vi "MatrixSwitch.vi"(8 "error in (no error)":errorcluster, 10 "Action":T1(ring), 11 "GPIBSwitching in":refnum<class "GPIBSwitching.lvclass">) -> (0 "error out":errorcluster, 3 "GPIBSwitching out":refnum<class "GPIBSwitching.lvclass">)   [LabVIEW 2018, in "GPIBSwitching.lvclass"]
uses:
  GPIBSwitching.lvclass
  InstrumentSetup.vi
  InstrControl.lvclass
panel:
  out "Display Matrix":bool[][](array[boolean])
  # "Pickering Matrix Settings"
  # "X1"
  # "X2"
  # "X3"
  # "X4"
  # "X5"
  # "X6"
  # "X7"
  # "X8"
  # "X9"
  # "X10"
  # "X11"
  # "X12"
  # "Y1"
  # "Y2"
  # "Y3"
  # "Y4"
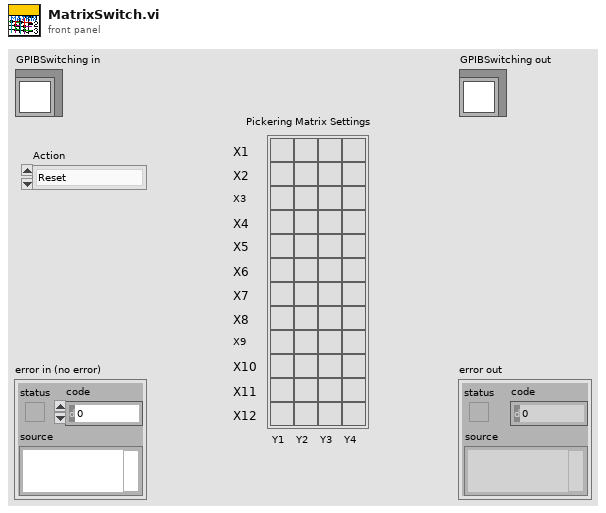
[diagram p1: front panel]
types:
  T1 = enum16{"Reset", "Ground", "Striptest SMU", "Striptest LCR", "IV", "CV", "Interstrip Cap", "Interstrip Res", "Setup StripTest"}
  T2 = cluster{"Matrix address":string, "Mux1 address":string, "Mux2 address":string, "Matrix used?":bool, "Switching":refnum<class "Switching.lvclass">, "Matrix X Channels":cluster{"Bias Supply / SMU LO":i32, "Bias Supply / SMU HI":i32, "CV Box LO":i32, "CV Box HI":i32, "CV Box LO IN":i32, "CV Box HI IN":i32, "Volt meter LO":i32, "Volt meter HI":i32, "Mux1 C1":i32, "Mux1 C2":i32, "Mux2 C1":i32, "Mux2 C2":i32}}
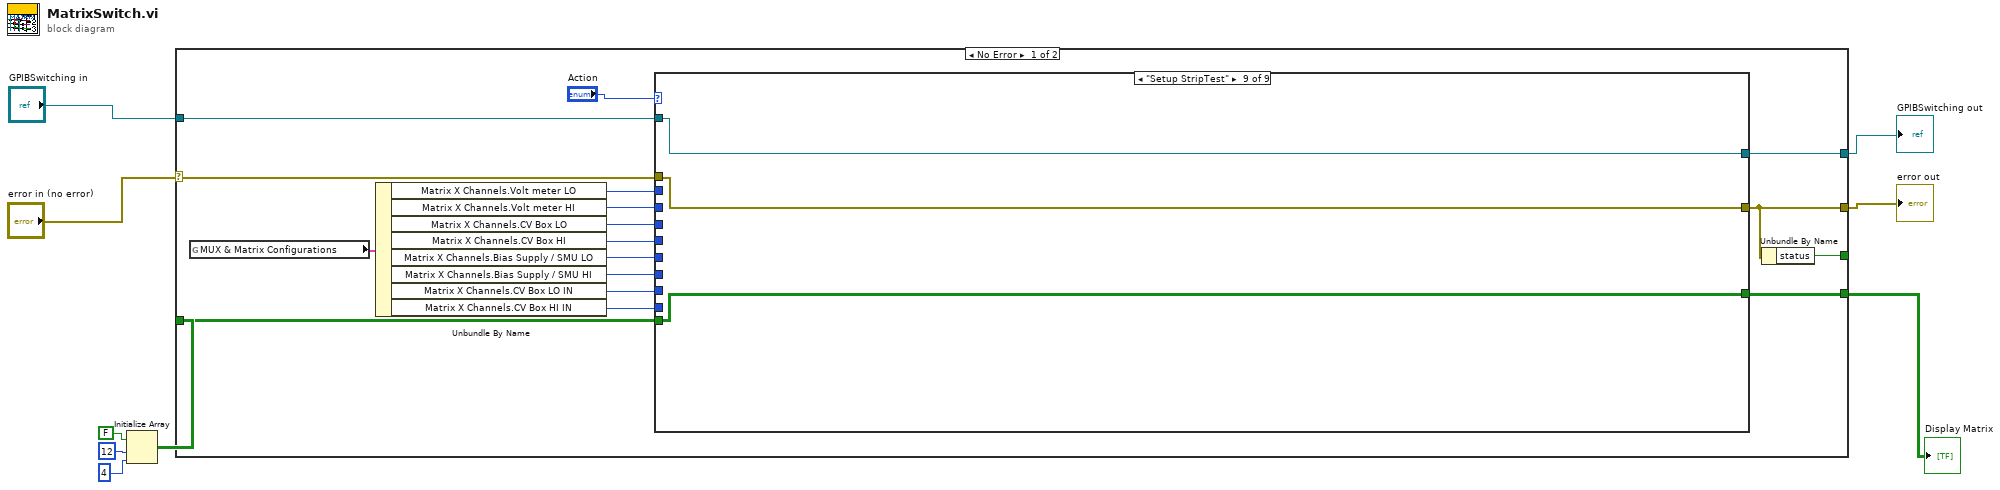
[diagram p0: block diagram]
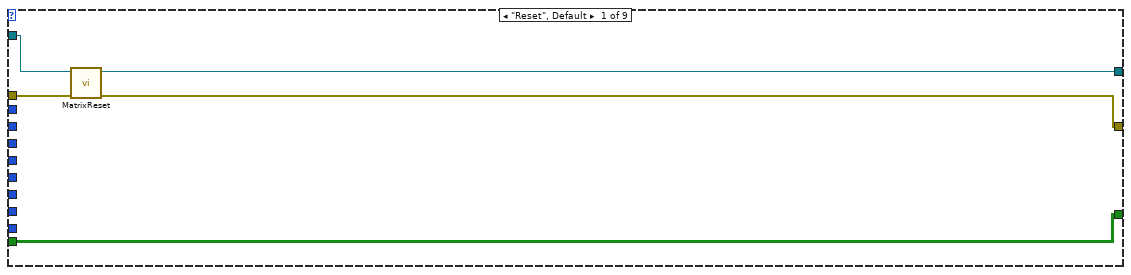
[diagram p2: hidden frame]
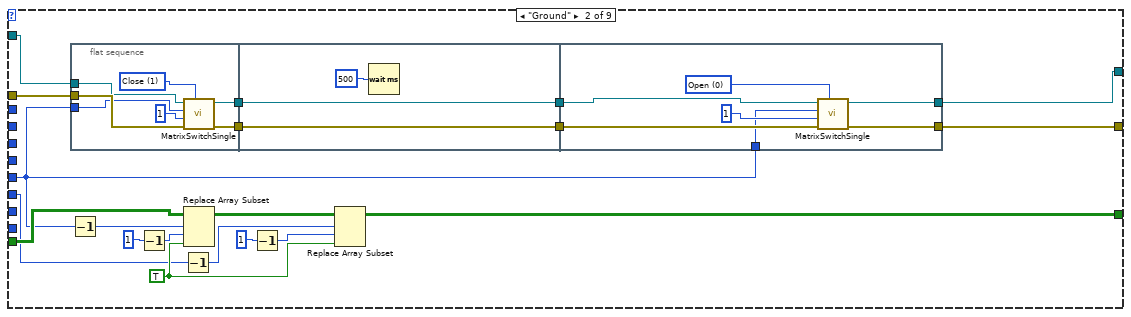
[diagram p3: hidden frame]
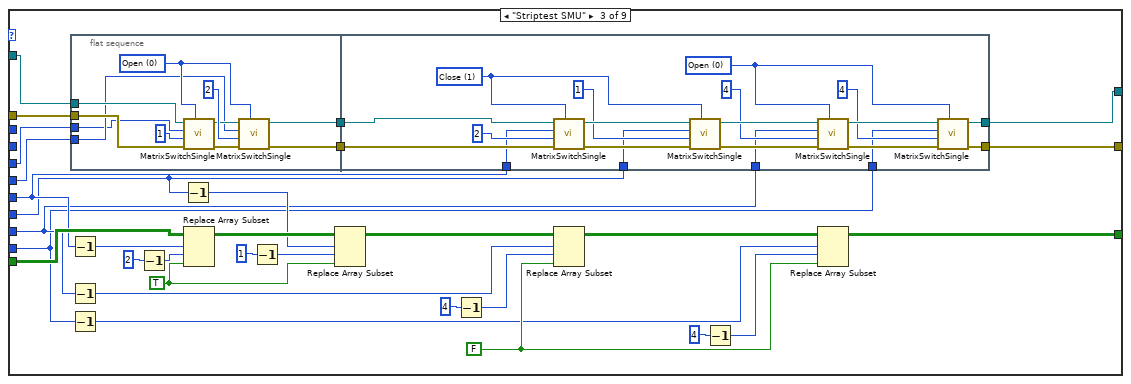
[diagram p4: hidden frame]
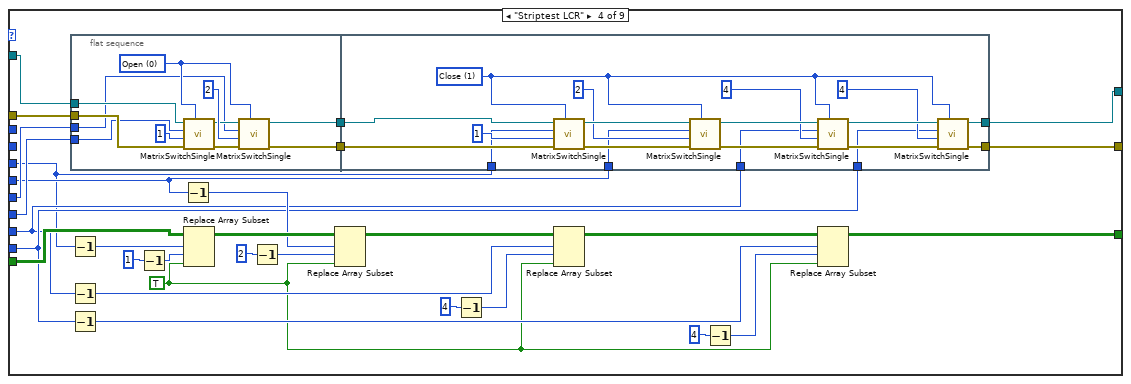
[diagram p5: hidden frame]
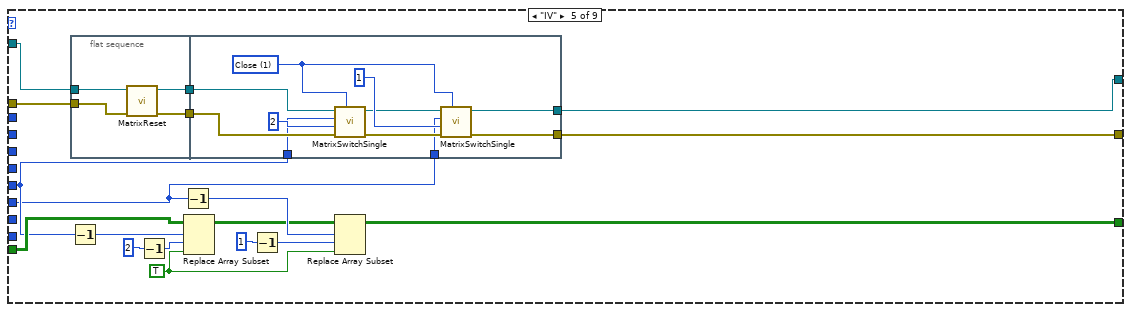
[diagram p6: hidden frame]
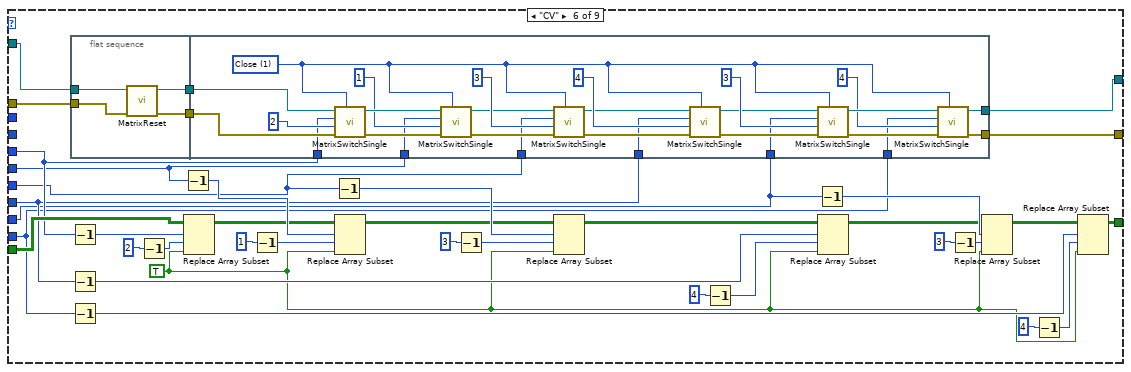
[diagram p7: hidden frame]
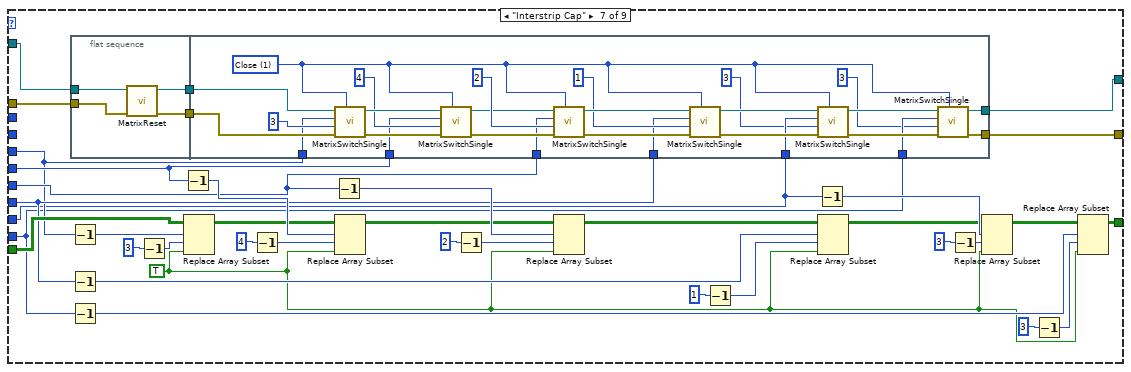
[diagram p8: hidden frame]
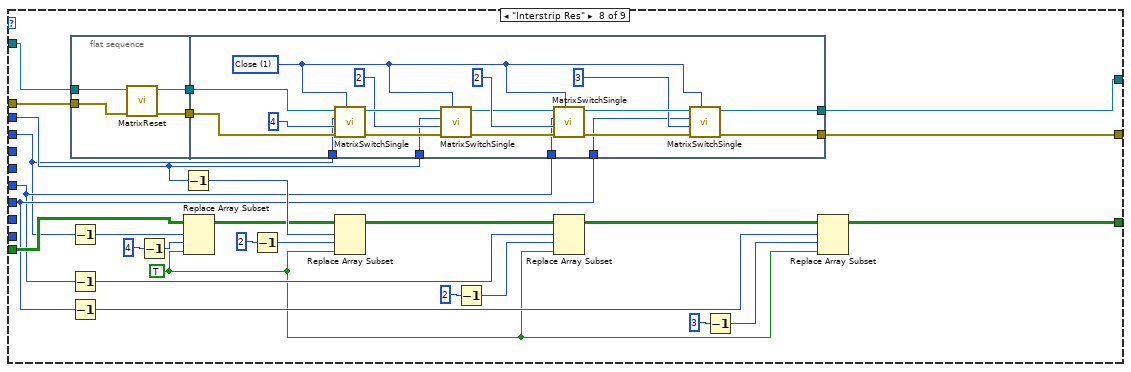
[diagram p9: hidden frame]
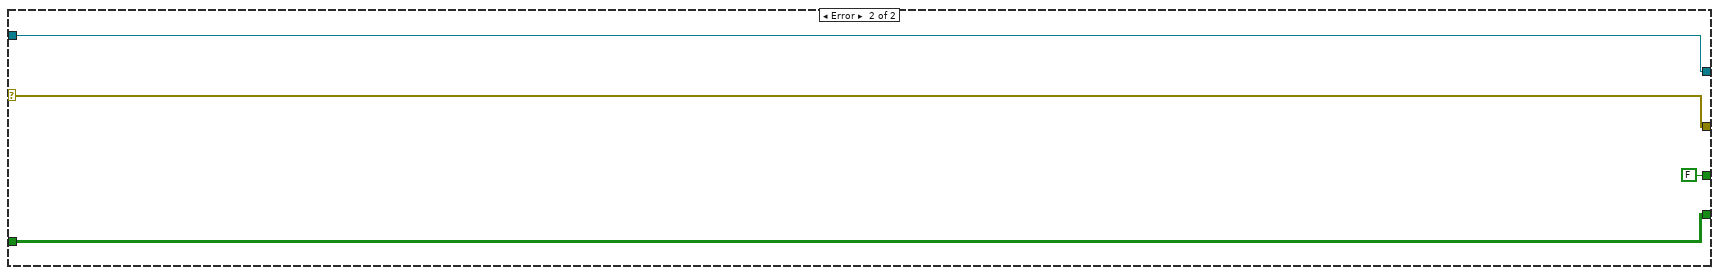
[diagram p10: hidden frame]
diagram:
  n1 = Initialize Array(FALSE, 12, 4) -> (w5:bool[][])
  n2 = case shown="No Error" "error in (no error)" {
    selector: "error in (no error)" -> [w20 w419]
    tunnel: [w23 w419] -> w3
    tunnel: [w24 w418] -> w4
    tunnel: "GPIBSwitching in" -> [w21 w418]
    tunnel: [w22 FALSE] -> _
    tunnel: w5 -> [w26 w416]
    tunnel: [w25 w416] -> w9
    frame No Error {
      n3 = global read "InstrumentSetup.vi" "MUX & Matrix Configurations"() -> (w19:T2)
      n4 = Unbundle By Name(w19) -> ("Matrix X Channels.Volt meter LO"=w13:i32, "Matrix X Channels.Volt meter HI"=w14:i32, "Matrix X Channels.CV Box LO"=w18:i32, "Matrix X Channels.CV Box HI"=w17:i32, "Matrix X Channels.Bias Supply / SMU LO"=w11:i32, "Matrix X Channels.Bias Supply / SMU HI"=w12:i32, "Matrix X Channels.CV Box LO IN"=w16:i32, "Matrix X Channels.CV Box HI IN"=w15:i32)
      n5 = case shown="\"Setup StripTest\"" "Action" {
        tunnel: w26 -> [w31 w36 w86 w149 w199 w236 w316 w374 w413]
        tunnel: [w31 w34 w85 w148 w200 w237 w293 w375 w413] -> w25
        tunnel: w20 -> [w28 w51 w75 w138 w207 w235 w315 w373 w414]
        tunnel: w21 -> [w30 w48 w77 w137 w208 w234 w314 w372 w415]
        tunnel: [w29 w45 w80 w143 w196 w230 w310 w368 w415] -> w24
        tunnel: [w27 w44 w79 w142 w195 w231 w311 w369 w414] -> w23
        tunnel: w11 -> [_ w33 w72 w135 w192 w227 w307 w364 _]
        tunnel: w12 -> [_ w32 w71 w136 w191 w226 w308 w365 _]
        tunnel: w18 -> [_ _ w73 w131 _ w229 w305 _ _]
        tunnel: w17 -> [_ _ w74 w132 _ w228 w306 _ _]
        tunnel: w16 -> [_ _ w70 w133 _ w225 w297 _ _]
        tunnel: w15 -> [_ _ w69 w134 _ w224 w296 _ _]
        tunnel: w13 -> [_ _ _ _ _ _ _ w363 _]
        tunnel: w14 -> [_ _ _ _ _ _ _ w362 _]
        frame "Reset", Default {
          n6 = call-dynamic "MatrixReset.vi"("error in (no error)"=w28, "GPIBSwitching in"=w30) -> ("error out"=w27:errorcluster, "GPIBSwitching out"=w29:refnum<class "GPIBSwitching.lvclass">)  [unwired: 8 in]
        }
        frame "Ground" {
          w42 = TRUE
          n7 = Decrement(x=w33) -> (x-1=w37:i32)
          n8 = flat-sequence {
            tunnel: w51 -> [w56]
            tunnel: [w55] -> w50
            tunnel: w48 -> [w54]
            tunnel: [w53] -> w46
            tunnel: w33 -> [w52]
            tunnel: w50 -> [w60]
            tunnel: [w60] -> w49
            tunnel: [w59] -> w47
            tunnel: w46 -> [w59]
            tunnel: w49 -> [w67]
            tunnel: w47 -> [w65]
            tunnel: [w64] -> w45
            tunnel: [w63] -> w44
            tunnel: w33 -> [w62]
            frame #0 {
              w58 = u16 1 items=["Open", "Close"] ("Switch action")
              n9 = call-dynamic "MatrixSwitchSingle.vi"("Switch action"=w58, "error in (no error)"=w56, "Matrix Y"=1, "Matrix X"=w52, "GPIBSwitching in"=w54) -> ("error out"=w55:errorcluster, "GPIBSwitching out"=w53:refnum<class "GPIBSwitching.lvclass">)  [unwired: 4 in, 1 out]
            }
            frame #1 {
              n10 = Wait (ms)(milliseconds to wait=u32 500) -> ()  [unwired: 1 out]
            }
            frame #2 {
              w68 = u16 0 items=["Open", "Close"] ("Switch action")
              n11 = call-dynamic "MatrixSwitchSingle.vi"("Switch action"=w68, "error in (no error)"=w67, "Matrix Y"=1, "Matrix X"=w62, "GPIBSwitching in"=w65) -> ("error out"=w63:errorcluster, "GPIBSwitching out"=w64:refnum<class "GPIBSwitching.lvclass">)  [unwired: 4 in, 1 out]
            }
          }
          n12 = Decrement(x=1 ("Matrix Y")) -> (x-1=w38:i32)
          n13 = Decrement(x=w32) -> (x-1=w39:i32)
          n14 = Replace Array Subset(array=w36, new element=w42, index (row)=w37, index (col)=w38) -> (w43:bool[][])
          n15 = Decrement(x=1 ("Matrix Y")) -> (x-1=w40:i32)
          n16 = Replace Array Subset(array=w43, new element=w42, index (row)=w39, index (col)=w40) -> (w34:bool[][])
        }
        frame "Striptest SMU" {
          w99 = FALSE
          w98 = TRUE
          n17 = Decrement(x=w72) -> (x-1=w88:i32)
          n18 = Decrement(x=w70) -> (x-1=w93:i32)
          n19 = Decrement(x=w69) -> (x-1=w94:i32)
          n20 = flat-sequence {
            tunnel: [w106] -> w78
            tunnel: w77 -> [w104]
            tunnel: [w103] -> w76
            tunnel: w75 -> [w102]
            tunnel: w74 -> [w101]
            tunnel: w73 -> [w100]
            tunnel: [w119] -> w80
            tunnel: [w118] -> w79
            tunnel: w78 -> [w116]
            tunnel: w76 -> [w115]
            tunnel: w70 -> [w114]
            tunnel: w69 -> [w113]
            tunnel: w71 -> [w112]
            tunnel: w72 -> [w111]
            frame #0 {
              w105 = u16 0 items=["Open", "Close"] ("Switch action")
              n21 = call-dynamic "MatrixSwitchSingle.vi"("Switch action"=w105, "error in (no error)"=w102, "Matrix Y"=1, "Matrix X"=w100, "GPIBSwitching in"=w104) -> ("error out"=w109:errorcluster, "GPIBSwitching out"=w108:refnum<class "GPIBSwitching.lvclass">)  [unwired: 4 in, 1 out]
              n22 = call-dynamic "MatrixSwitchSingle.vi"("Switch action"=w105, "error in (no error)"=w109, "Matrix Y"=2, "Matrix X"=w101, "GPIBSwitching in"=w108) -> ("error out"=w106:errorcluster, "GPIBSwitching out"=w103:refnum<class "GPIBSwitching.lvclass">)  [unwired: 4 in, 1 out]
            }
            frame #1 {
              w117 = u16 0 items=["Open", "Close"] ("Switch action")
              w128 = u16 1 items=["Open", "Close"] ("Switch action")
              n23 = call-dynamic "MatrixSwitchSingle.vi"("Switch action"=w128, "error in (no error)"=w116, "Matrix Y"=2, "Matrix X"=w111, "GPIBSwitching in"=w115) -> ("error out"=w126:errorcluster, "GPIBSwitching out"=w129:refnum<class "GPIBSwitching.lvclass">)  [unwired: 4 in, 1 out]
              n24 = call-dynamic "MatrixSwitchSingle.vi"("Switch action"=w128, "error in (no error)"=w126, "Matrix Y"=1, "Matrix X"=w112, "GPIBSwitching in"=w129) -> ("error out"=w124:errorcluster, "GPIBSwitching out"=w125:refnum<class "GPIBSwitching.lvclass">)  [unwired: 4 in, 1 out]
              n25 = call-dynamic "MatrixSwitchSingle.vi"("Switch action"=w117, "error in (no error)"=w124, "Matrix Y"=4, "Matrix X"=w114, "GPIBSwitching in"=w125) -> ("error out"=w121:errorcluster, "GPIBSwitching out"=w122:refnum<class "GPIBSwitching.lvclass">)  [unwired: 4 in, 1 out]
              n26 = call-dynamic "MatrixSwitchSingle.vi"("Switch action"=w117, "error in (no error)"=w121, "Matrix Y"=4, "Matrix X"=w113, "GPIBSwitching in"=w122) -> ("error out"=w118:errorcluster, "GPIBSwitching out"=w119:refnum<class "GPIBSwitching.lvclass">)  [unwired: 4 in, 1 out]
            }
          }
          n27 = Decrement(x=2 ("Matrix Y")) -> (x-1=w87:i32)
          n28 = Decrement(x=w71) -> (x-1=w89:i32)
          n29 = Replace Array Subset(array=w86, new element=w98, index (row)=w88, index (col)=w87) -> (w91:bool[][])
          n30 = Decrement(x=1 ("Matrix Y")) -> (x-1=w90:i32)
          n31 = Replace Array Subset(array=w91, new element=w98, index (row)=w89, index (col)=w90) -> (w97:bool[][])
          n32 = Decrement(x=4 ("Matrix Y")) -> (x-1=w92:i32)
          n33 = Replace Array Subset(array=w97, new element=w99, index (row)=w93, index (col)=w92) -> (w96:bool[][])
          n34 = Decrement(x=4 ("Matrix Y")) -> (x-1=w95:i32)
          n35 = Replace Array Subset(array=w96, new element=w99, index (row)=w94, index (col)=w95) -> (w85:bool[][])
        }
        frame "Striptest LCR" {
          w141 = TRUE
          n36 = Decrement(x=w131) -> (x-1=w151:i32)
          n37 = Decrement(x=w133) -> (x-1=w156:i32)
          n38 = Decrement(x=w134) -> (x-1=w157:i32)
          n39 = flat-sequence {
            tunnel: [w167] -> w140
            tunnel: [w166] -> w139
            tunnel: w138 -> [w165]
            tunnel: w137 -> [w164]
            tunnel: w135 -> [w162]
            tunnel: w136 -> [w161]
            tunnel: [w180] -> w143
            tunnel: [w179] -> w142
            tunnel: w140 -> [w177]
            tunnel: w139 -> [w176]
            tunnel: w131 -> [w175]
            tunnel: w132 -> [w174]
            tunnel: w133 -> [w173]
            tunnel: w134 -> [w172]
            frame #0 {
              w163 = u16 0 items=["Open", "Close"] ("Switch action")
              n40 = call-dynamic "MatrixSwitchSingle.vi"("Switch action"=w163, "error in (no error)"=w165, "Matrix Y"=1, "Matrix X"=w161, "GPIBSwitching in"=w164) -> ("error out"=w170:errorcluster, "GPIBSwitching out"=w169:refnum<class "GPIBSwitching.lvclass">)  [unwired: 4 in, 1 out]
              n41 = call-dynamic "MatrixSwitchSingle.vi"("Switch action"=w163, "error in (no error)"=w170, "Matrix Y"=2, "Matrix X"=w162, "GPIBSwitching in"=w169) -> ("error out"=w166:errorcluster, "GPIBSwitching out"=w167:refnum<class "GPIBSwitching.lvclass">)  [unwired: 4 in, 1 out]
            }
            frame #1 {
              w178 = u16 1 items=["Open", "Close"] ("Switch action")
              n42 = call-dynamic "MatrixSwitchSingle.vi"("Switch action"=w178, "error in (no error)"=w176, "Matrix Y"=1, "Matrix X"=w175, "GPIBSwitching in"=w177) -> ("error out"=w187:errorcluster, "GPIBSwitching out"=w189:refnum<class "GPIBSwitching.lvclass">)  [unwired: 4 in, 1 out]
              n43 = call-dynamic "MatrixSwitchSingle.vi"("Switch action"=w178, "error in (no error)"=w187, "Matrix Y"=2, "Matrix X"=w174, "GPIBSwitching in"=w189) -> ("error out"=w185:errorcluster, "GPIBSwitching out"=w186:refnum<class "GPIBSwitching.lvclass">)  [unwired: 4 in, 1 out]
              n44 = call-dynamic "MatrixSwitchSingle.vi"("Switch action"=w178, "error in (no error)"=w185, "Matrix Y"=4, "Matrix X"=w173, "GPIBSwitching in"=w186) -> ("error out"=w182:errorcluster, "GPIBSwitching out"=w183:refnum<class "GPIBSwitching.lvclass">)  [unwired: 4 in, 1 out]
              n45 = call-dynamic "MatrixSwitchSingle.vi"("Switch action"=w178, "error in (no error)"=w182, "Matrix Y"=4, "Matrix X"=w172, "GPIBSwitching in"=w183) -> ("error out"=w179:errorcluster, "GPIBSwitching out"=w180:refnum<class "GPIBSwitching.lvclass">)  [unwired: 4 in, 1 out]
            }
          }
          n46 = Decrement(x=1 ("Matrix Y")) -> (x-1=w150:i32)
          n47 = Decrement(x=w132) -> (x-1=w152:i32)
          n48 = Replace Array Subset(array=w149, new element=w141, index (row)=w151, index (col)=w150) -> (w154:bool[][])
          n49 = Decrement(x=2 ("Matrix Y")) -> (x-1=w153:i32)
          n50 = Replace Array Subset(array=w154, new element=w141, index (row)=w152, index (col)=w153) -> (w160:bool[][])
          n51 = Decrement(x=4 ("Matrix Y")) -> (x-1=w155:i32)
          n52 = Replace Array Subset(array=w160, new element=w141, index (row)=w156, index (col)=w155) -> (w159:bool[][])
          n53 = Decrement(x=4 ("Matrix Y")) -> (x-1=w158:i32)
          n54 = Replace Array Subset(array=w159, new element=w141, index (row)=w157, index (col)=w158) -> (w148:bool[][])
        }
        frame "IV" {
          w202 = TRUE
          n55 = Decrement(x=w192) -> (x-1=w204:i32)
          n56 = flat-sequence {
            tunnel: w208 -> [w212]
            tunnel: w207 -> [w211]
            tunnel: [w210] -> w198
            tunnel: [w209] -> w197
            tunnel: w198 -> [w218]
            tunnel: w197 -> [w217]
            tunnel: [w216] -> w196
            tunnel: [w215] -> w195
            tunnel: w191 -> [w214]
            tunnel: w192 -> [w213]
            frame #0 {
              n57 = call-dynamic "MatrixReset.vi"("error in (no error)"=w211, "GPIBSwitching in"=w212) -> ("error out"=w209:errorcluster, "GPIBSwitching out"=w210:refnum<class "GPIBSwitching.lvclass">)  [unwired: 8 in]
            }
            frame #1 {
              w223 = u16 1 items=["Open", "Close"] ("Switch action")
              n58 = call-dynamic "MatrixSwitchSingle.vi"("Switch action"=w223, "error in (no error)"=w217, "Matrix Y"=2, "Matrix X"=w213, "GPIBSwitching in"=w218) -> ("error out"=w221:errorcluster, "GPIBSwitching out"=w220:refnum<class "GPIBSwitching.lvclass">)  [unwired: 4 in, 1 out]
              n59 = call-dynamic "MatrixSwitchSingle.vi"("Switch action"=w223, "error in (no error)"=w221, "Matrix Y"=1, "Matrix X"=w214, "GPIBSwitching in"=w220) -> ("error out"=w215:errorcluster, "GPIBSwitching out"=w216:refnum<class "GPIBSwitching.lvclass">)  [unwired: 4 in, 1 out]
            }
          }
          n60 = Decrement(x=2 ("Matrix Y")) -> (x-1=w203:i32)
          n61 = Decrement(x=w191) -> (x-1=w206:i32)
          n62 = Replace Array Subset(array=w199, new element=w202, index (row)=w204, index (col)=w203) -> (w201:bool[][])
          n63 = Decrement(x=1 ("Matrix Y")) -> (x-1=w205:i32)
          n64 = Replace Array Subset(array=w201, new element=w202, index (row)=w206, index (col)=w205) -> (w200:bool[][])
        }
        frame "CV" {
          w246 = TRUE
          n65 = Decrement(x=w229) -> (x-1=w259:i32)
          n66 = Decrement(x=w226) -> (x-1=w252:i32)
          n67 = Decrement(x=w224) -> (x-1=w251:i32)
          n68 = flat-sequence {
            tunnel: w235 -> [w265]
            tunnel: w234 -> [w264]
            tunnel: [w263] -> w233
            tunnel: [w262] -> w232
            tunnel: w233 -> [w275]
            tunnel: w232 -> [w274]
            tunnel: [w273] -> w231
            tunnel: [w272] -> w230
            tunnel: w229 -> [w271]
            tunnel: w228 -> [w270]
            tunnel: w227 -> [w269]
            tunnel: w226 -> [w268]
            tunnel: w225 -> [w267]
            tunnel: w224 -> [w266]
            frame #0 {
              n69 = call-dynamic "MatrixReset.vi"("error in (no error)"=w265, "GPIBSwitching in"=w264) -> ("error out"=w262:errorcluster, "GPIBSwitching out"=w263:refnum<class "GPIBSwitching.lvclass">)  [unwired: 8 in]
            }
            frame #1 {
              w278 = u16 1 items=["Open", "Close"] ("Switch action")
              n70 = call-dynamic "MatrixSwitchSingle.vi"("Switch action"=w278, "error in (no error)"=w274, "Matrix Y"=2, "Matrix X"=w271, "GPIBSwitching in"=w275) -> ("error out"=w280:errorcluster, "GPIBSwitching out"=w281:refnum<class "GPIBSwitching.lvclass">)  [unwired: 4 in, 1 out]
              n71 = call-dynamic "MatrixSwitchSingle.vi"("Switch action"=w278, "error in (no error)"=w280, "Matrix Y"=1, "Matrix X"=w270, "GPIBSwitching in"=w281) -> ("error out"=w276:errorcluster, "GPIBSwitching out"=w277:refnum<class "GPIBSwitching.lvclass">)  [unwired: 4 in, 1 out]
              n72 = call-dynamic "MatrixSwitchSingle.vi"("Switch action"=w278, "error in (no error)"=w276, "Matrix Y"=3, "Matrix X"=w269, "GPIBSwitching in"=w277) -> ("error out"=w291:errorcluster, "GPIBSwitching out"=w290:refnum<class "GPIBSwitching.lvclass">)  [unwired: 4 in, 1 out]
              n73 = call-dynamic "MatrixSwitchSingle.vi"("Switch action"=w278, "error in (no error)"=w291, "Matrix Y"=4, "Matrix X"=w268, "GPIBSwitching in"=w290) -> ("error out"=w283:errorcluster, "GPIBSwitching out"=w284:refnum<class "GPIBSwitching.lvclass">)  [unwired: 4 in, 1 out]
              n74 = call-dynamic "MatrixSwitchSingle.vi"("Switch action"=w278, "error in (no error)"=w283, "Matrix Y"=3, "Matrix X"=w267, "GPIBSwitching in"=w284) -> ("error out"=w286:errorcluster, "GPIBSwitching out"=w287:refnum<class "GPIBSwitching.lvclass">)  [unwired: 4 in, 1 out]
              n75 = call-dynamic "MatrixSwitchSingle.vi"("Switch action"=w278, "error in (no error)"=w286, "Matrix Y"=4, "Matrix X"=w266, "GPIBSwitching in"=w287) -> ("error out"=w273:errorcluster, "GPIBSwitching out"=w272:refnum<class "GPIBSwitching.lvclass">)  [unwired: 4 in, 1 out]
            }
          }
          n76 = Decrement(x=2 ("Matrix Y")) -> (x-1=w258:i32)
          n77 = Decrement(x=w228) -> (x-1=w261:i32)
          n78 = Replace Array Subset(array=w236, new element=w246, index (row)=w259, index (col)=w258) -> (w257:bool[][])
          n79 = Decrement(x=1 ("Matrix Y")) -> (x-1=w260:i32)
          n80 = Decrement(x=w227) -> (x-1=w254:i32)
          n81 = Replace Array Subset(array=w257, new element=w246, index (row)=w261, index (col)=w260) -> (w239:bool[][])
          n82 = Decrement(x=3 ("Matrix Y")) -> (x-1=w255:i32)
          n83 = Replace Array Subset(array=w239, new element=w246, index (row)=w254, index (col)=w255) -> (w256:bool[][])
          n84 = Decrement(x=4 ("Matrix Y")) -> (x-1=w253:i32)
          n85 = Decrement(x=w225) -> (x-1=w249:i32)
          n86 = Replace Array Subset(array=w256, new element=w246, index (row)=w252, index (col)=w253) -> (w238:bool[][])
          n87 = Decrement(x=3 ("Matrix Y")) -> (x-1=w248:i32)
          n88 = Replace Array Subset(array=w238, new element=w246, index (row)=w249, index (col)=w248) -> (w247:bool[][])
          n89 = Decrement(x=4 ("Matrix Y")) -> (x-1=w250:i32)
          n90 = Replace Array Subset(array=w247, new element=w246, index (row)=w251, index (col)=w250) -> (w237:bool[][])
        }
        frame "Interstrip Cap" {
          w298 = TRUE
          n91 = Decrement(x=w305) -> (x-1=w328:i32)
          n92 = Decrement(x=w308) -> (x-1=w325:i32)
          n93 = Decrement(x=w296) -> (x-1=w304:i32)
          n94 = flat-sequence {
            tunnel: w315 -> [w334]
            tunnel: w314 -> [w333]
            tunnel: [w332] -> w313
            tunnel: [w331] -> w312
            tunnel: w313 -> [w353]
            tunnel: w312 -> [w352]
            tunnel: [w337] -> w311
            tunnel: [w336] -> w310
            tunnel: w305 -> [w349]
            tunnel: w306 -> [w348]
            tunnel: w307 -> [w347]
            tunnel: w308 -> [w346]
            tunnel: w297 -> [w341]
            tunnel: w296 -> [w340]
            frame #0 {
              n95 = call-dynamic "MatrixReset.vi"("error in (no error)"=w334, "GPIBSwitching in"=w333) -> ("error out"=w331:errorcluster, "GPIBSwitching out"=w332:refnum<class "GPIBSwitching.lvclass">)  [unwired: 8 in]
            }
            frame #1 {
              w335 = u16 1 items=["Open", "Close"] ("Switch action")
              n96 = call-dynamic "MatrixSwitchSingle.vi"("Switch action"=w335, "error in (no error)"=w352, "Matrix Y"=3, "Matrix X"=w349, "GPIBSwitching in"=w353) -> ("error out"=w355:errorcluster, "GPIBSwitching out"=w356:refnum<class "GPIBSwitching.lvclass">)  [unwired: 4 in, 1 out]
              n97 = call-dynamic "MatrixSwitchSingle.vi"("Switch action"=w335, "error in (no error)"=w355, "Matrix Y"=4, "Matrix X"=w348, "GPIBSwitching in"=w356) -> ("error out"=w350:errorcluster, "GPIBSwitching out"=w351:refnum<class "GPIBSwitching.lvclass">)  [unwired: 4 in, 1 out]
              n98 = call-dynamic "MatrixSwitchSingle.vi"("Switch action"=w335, "error in (no error)"=w350, "Matrix Y"=2, "Matrix X"=w347, "GPIBSwitching in"=w351) -> ("error out"=w359:errorcluster, "GPIBSwitching out"=w360:refnum<class "GPIBSwitching.lvclass">)  [unwired: 4 in, 1 out]
              n99 = call-dynamic "MatrixSwitchSingle.vi"("Switch action"=w335, "error in (no error)"=w359, "Matrix Y"=1, "Matrix X"=w346, "GPIBSwitching in"=w360) -> ("error out"=w343:errorcluster, "GPIBSwitching out"=w342:refnum<class "GPIBSwitching.lvclass">)  [unwired: 4 in, 1 out]
              n100 = call-dynamic "MatrixSwitchSingle.vi"("Switch action"=w335, "error in (no error)"=w343, "Matrix Y"=3, "Matrix X"=w341, "GPIBSwitching in"=w342) -> ("error out"=w345:errorcluster, "GPIBSwitching out"=w344:refnum<class "GPIBSwitching.lvclass">)  [unwired: 4 in, 1 out]
              n101 = call-dynamic "MatrixSwitchSingle.vi"("Switch action"=w335, "error in (no error)"=w345, "Matrix Y"=3, "Matrix X"=w340, "GPIBSwitching in"=w344) -> ("error out"=w337:errorcluster, "GPIBSwitching out"=w336:refnum<class "GPIBSwitching.lvclass">)  [unwired: 4 in, 1 out]
            }
          }
          n102 = Decrement(x=3 ("Matrix Y")) -> (x-1=w327:i32)
          n103 = Decrement(x=w306) -> (x-1=w330:i32)
          n104 = Replace Array Subset(array=w316, new element=w298, index (row)=w328, index (col)=w327) -> (w326:bool[][])
          n105 = Decrement(x=4 ("Matrix Y")) -> (x-1=w329:i32)
          n106 = Decrement(x=w307) -> (x-1=w323:i32)
          n107 = Replace Array Subset(array=w326, new element=w298, index (row)=w330, index (col)=w329) -> (w309:bool[][])
          n108 = Decrement(x=2 ("Matrix Y")) -> (x-1=w322:i32)
          n109 = Replace Array Subset(array=w309, new element=w298, index (row)=w323, index (col)=w322) -> (w321:bool[][])
          n110 = Decrement(x=1 ("Matrix Y")) -> (x-1=w324:i32)
          n111 = Decrement(x=w297) -> (x-1=w302:i32)
          n112 = Replace Array Subset(array=w321, new element=w298, index (row)=w325, index (col)=w324) -> (w300:bool[][])
          n113 = Decrement(x=3 ("Matrix Y")) -> (x-1=w301:i32)
          n114 = Replace Array Subset(array=w300, new element=w298, index (row)=w302, index (col)=w301) -> (w299:bool[][])
          n115 = Decrement(x=3 ("Matrix Y")) -> (x-1=w303:i32)
          n116 = Replace Array Subset(array=w299, new element=w298, index (row)=w304, index (col)=w303) -> (w293:bool[][])
        }
        frame "Interstrip Res" {
          w366 = TRUE
          n117 = Decrement(x=w362) -> (x-1=w387:i32)
          n118 = Decrement(x=w364) -> (x-1=w382:i32)
          n119 = Decrement(x=w365) -> (x-1=w384:i32)
          n120 = flat-sequence {
            tunnel: w373 -> [w393]
            tunnel: w372 -> [w392]
            tunnel: [w391] -> w371
            tunnel: [w390] -> w370
            tunnel: w371 -> [w403]
            tunnel: w370 -> [w402]
            tunnel: [w401] -> w369
            tunnel: [w400] -> w368
            tunnel: w364 -> [w397]
            tunnel: w365 -> [w396]
            tunnel: w363 -> [w395]
            tunnel: w362 -> [w394]
            frame #0 {
              n121 = call-dynamic "MatrixReset.vi"("error in (no error)"=w393, "GPIBSwitching in"=w392) -> ("error out"=w390:errorcluster, "GPIBSwitching out"=w391:refnum<class "GPIBSwitching.lvclass">)  [unwired: 8 in]
            }
            frame #1 {
              w404 = u16 1 items=["Open", "Close"] ("Switch action")
              n122 = call-dynamic "MatrixSwitchSingle.vi"("Switch action"=w404, "error in (no error)"=w402, "Matrix Y"=4, "Matrix X"=w394, "GPIBSwitching in"=w403) -> ("error out"=w406:errorcluster, "GPIBSwitching out"=w407:refnum<class "GPIBSwitching.lvclass">)  [unwired: 4 in, 1 out]
              n123 = call-dynamic "MatrixSwitchSingle.vi"("Switch action"=w404, "error in (no error)"=w406, "Matrix Y"=2, "Matrix X"=w395, "GPIBSwitching in"=w407) -> ("error out"=w398:errorcluster, "GPIBSwitching out"=w399:refnum<class "GPIBSwitching.lvclass">)  [unwired: 4 in, 1 out]
              n124 = call-dynamic "MatrixSwitchSingle.vi"("Switch action"=w404, "error in (no error)"=w398, "Matrix Y"=2, "Matrix X"=w397, "GPIBSwitching in"=w399) -> ("error out"=w410:errorcluster, "GPIBSwitching out"=w411:refnum<class "GPIBSwitching.lvclass">)  [unwired: 4 in, 1 out]
              n125 = call-dynamic "MatrixSwitchSingle.vi"("Switch action"=w404, "error in (no error)"=w410, "Matrix Y"=3, "Matrix X"=w396, "GPIBSwitching in"=w411) -> ("error out"=w401:errorcluster, "GPIBSwitching out"=w400:refnum<class "GPIBSwitching.lvclass">)  [unwired: 4 in, 1 out]
            }
          }
          n126 = Decrement(x=4 ("Matrix Y")) -> (x-1=w386:i32)
          n127 = Decrement(x=w363) -> (x-1=w389:i32)
          n128 = Replace Array Subset(array=w374, new element=w366, index (row)=w387, index (col)=w386) -> (w385:bool[][])
          n129 = Decrement(x=2 ("Matrix Y")) -> (x-1=w388:i32)
          n130 = Replace Array Subset(array=w385, new element=w366, index (row)=w389, index (col)=w388) -> (w367:bool[][])
          n131 = Decrement(x=2 ("Matrix Y")) -> (x-1=w381:i32)
          n132 = Replace Array Subset(array=w367, new element=w366, index (row)=w382, index (col)=w381) -> (w380:bool[][])
          n133 = Decrement(x=3 ("Matrix Y")) -> (x-1=w383:i32)
          n134 = Replace Array Subset(array=w380, new element=w366, index (row)=w384, index (col)=w383) -> (w375:bool[][])
        }
        frame "Setup StripTest" {
        }
      }
      n135 = Unbundle By Name(w23) -> ("status"=w22:bool)
    }
    frame Error {
    }
  }
  "error out" <- w3
  "GPIBSwitching out" <- w4
  "Display Matrix" <- w9
